vi "Write SequenceIndices.vi"(8 "error in (no error)":errorcluster, 10 "SequenceIndices":refnum<class "SequenceIndex.lvclass">[](array[class]), 11 "VariableManager in":refnum<class "VariableManager.lvclass">) -> (0 "error out":errorcluster, 3 "VariableManager out":refnum<class "VariableManager.lvclass">)   [LabVIEW 2013, in "VariableManager.lvclass"]
uses:
  VariableManager.lvclass
  SequenceIndex/SequenceIndex.lvclass
  VariableManager.lvclass/VariableManager.ctl
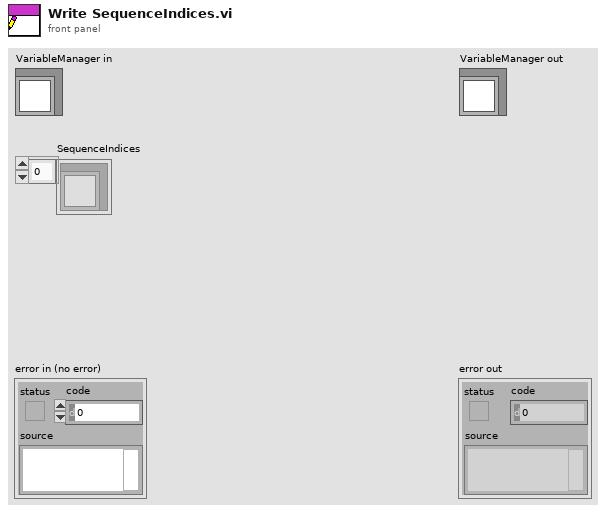
[diagram p1: front panel]
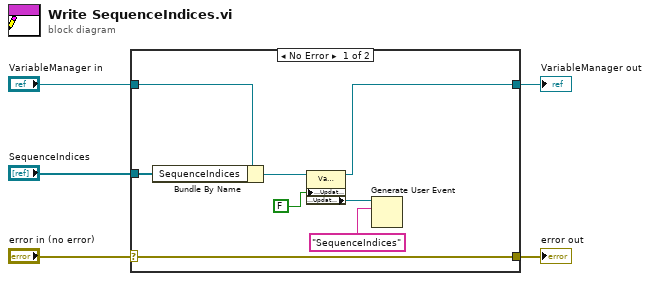
[diagram p0: block diagram]
diagram:
  n1 = case shown="No Error" "error in (no error)" {
    selector: "error in (no error)" -> [w13 w14]
    tunnel: [w13 w14] -> w4
    tunnel: [w9 w15] -> w2
    tunnel: "VariableManager in" -> [w12 w15]
    tunnel: "SequenceIndices" -> [w11 _]
    frame No Error {
      n2 = Bundle By Name(cluster=w12, "SequenceIndices"=w11) -> (w10:refnum<class "VariableManager.lvclass">)
      n3 = property class="VariableManager.lvclass"(reference=w10, "Accessors:UpdatedValues"=FALSE ("UpdatedValues")) -> (reference out=w9:refnum<class "VariableManager.lvclass">, "Accessors:UpdateEvent"=w7:refnum<user-event>)  [unwired: 1 in, 1 out]
      n4 = Generate User Event(user event=w7, event data cluster="SequenceIndices") -> ()  [unwired: 2 in, 2 out]
    }
    frame Error {
    }
  }
  "error out" <- w4
  "VariableManager out" <- w2
